vi "Analog Edge Trigger.vi"(8 "error in (no error)":errorcluster, 11 "4300 in":refnum<class "4300.lvclass">) -> (0 "error out":errorcluster, 3 "4300 out":refnum<class "4300.lvclass">)   [LabVIEW 2019, in "4300.lvlib" / "4300.lvclass"]
uses:
  Library/4300.lvclass
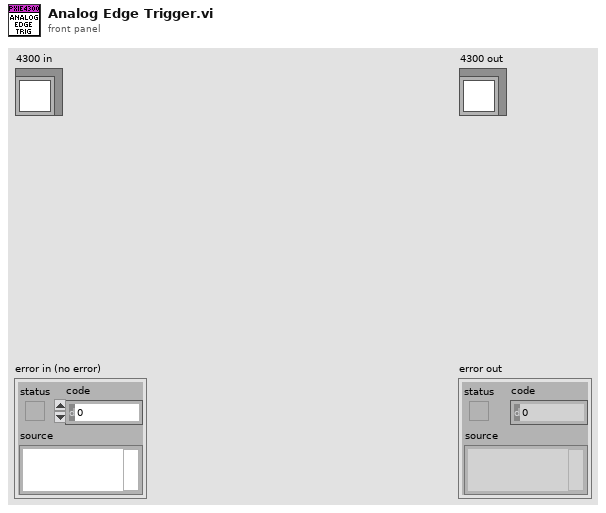
[diagram p1: front panel]
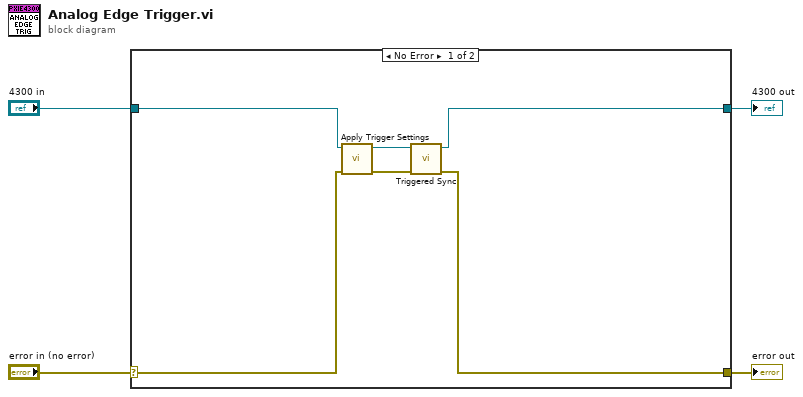
[diagram p0: block diagram]
diagram:
  n1 = case shown="No Error" "error in (no error)" {
    selector: "error in (no error)" -> [w6 w12]
    tunnel: [w5 w12] -> w3
    tunnel: [w7 w11] -> w1
    tunnel: "4300 in" -> [w8 w11]
    frame No Error {
      n2 = call-dynamic "Apply Trigger Settings.vi"("error in"=w6, "4300 in"=w8) -> ("error out"=w10:errorcluster, "4300 out"=w9:refnum<class "4300.lvclass">)  [unwired: 8 in]
      n3 = call "Triggered Sync.vi"("error in"=w10, "4300 in"=w9) -> ("error out"=w5:errorcluster, "4300 out"=w7:refnum<class "4300.lvclass">)  [unwired: 8 in]
    }
    frame Error {
    }
  }
  "error out" <- w3
  "4300 out" <- w1
